vi "Initialize.vi"(8 "error in (no error)":errorcluster, 10 "Angle-Value Pairs":T1[](array[typedef]), 11 "LinearInterpolation in":refnum<class "LinearInterpolation.lvclass">) -> (0 "error out":errorcluster, 3 "LinearInterpolation out":refnum<class "LinearInterpolation.lvclass">)   [LabVIEW 2011, in "LinearInterpolation.lvclass"]
uses:
  LinearInterpolation.lvclass
  AngleValuePair.ctl
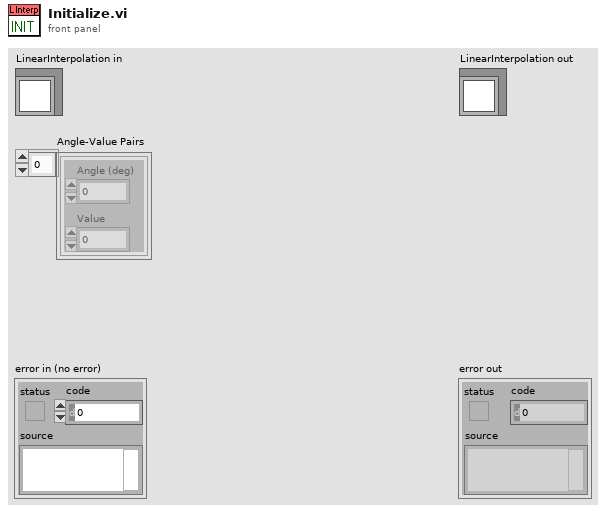
[diagram p1: front panel]
types:
  T1 = typedef "AngleValuePair.ctl" = cluster{"Angle (deg)":dbl, "Value":dbl}
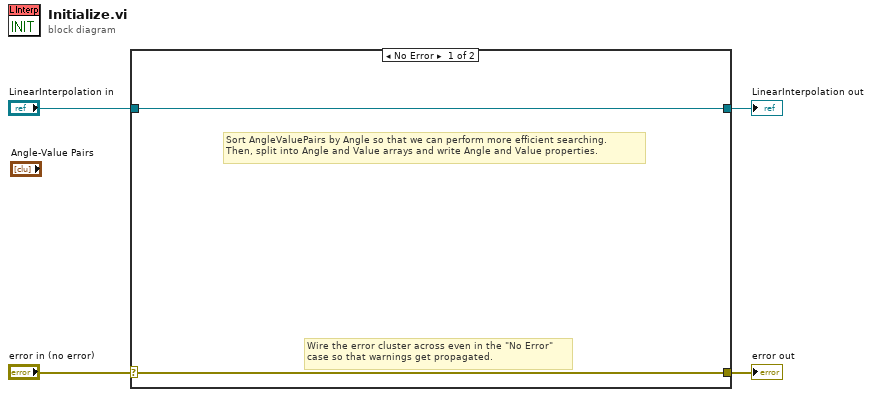
[diagram p0: block diagram]
diagram:
  n1 = case shown="No Error" "error in (no error)" {
    selector: "error in (no error)" -> [w5 w8]
    tunnel: [w5 w8] -> w3
    tunnel: [w6 w7] -> w1
    tunnel: "LinearInterpolation in" -> [w6 w7]
    frame No Error {
      # "Sort AngleValuePairs by Angle so that we can perform more efficient searching.\nThen, split into Angle and Value arrays and write Angle and Value properties."
      # "Wire the error cluster across even in the \"No Error\"\ncase so that warnings get propagated."
    }
    frame Error {
    }
  }
  "error out" <- w3
  "LinearInterpolation out" <- w1
